vi "LabVIEW RFID.vi"() -> ()   [LabVIEW 2010]
uses:
  <vilib>/Instr/_visa.llb/VISA Configure Serial Port (Instr).vi
  <vilib>/Utility/file.llb/Read From Spreadsheet File (I64).vi
  <vilib>/Utility/file.llb/Read From Spreadsheet File (string).vi
  <vilib>/Utility/file.llb/Write To Spreadsheet File (string).vi
  <vilib>/Utility/file.llb/Write To Spreadsheet File (I64).vi
panel:
  out "var":bool
  in  "Abrir Cacifo a partir de PC":bool
  in  "Endereço de Cacifo a abrir a partir de PC":dbl
  in  "Inserir novo utilizador/dar acesso a cacifo e atualizar base de dados":bool
  in  "default (0 I32)":u64
  in  "Pessoa a retirar acesso":string
  in  "Retirar acesso a cacifo e atualizar base de dasos":bool
  out "Enviado":string
  in  "Endereço do Cacifo a adicionar/remover":dbl
  out "Nomes":string[][](array[string])
  in  "Nome do novo utilizador":string
  out "Qual o utilizador?":string
  out "Código recebido":string
  out "Envia quando encontra 'a'":string
  out "Base de dados":i64[][](array[numeric])
  out "Matriz 2D":i64[][](array[numeric])
  out "Endereço do cacifo":u64
  out "Número de série do cartão":u64
  in  "VISA Resource Name":refnum<visa-resource-name>
  in  "stop":bool
  # "Adicionar utilizador e dar acesso a cacifos"
  # "Dados Recebidos na Porta Série"
  # "Retirar acesso de um utilizador a determinado cacifo"
  # "Reconhecimento de utilizador"
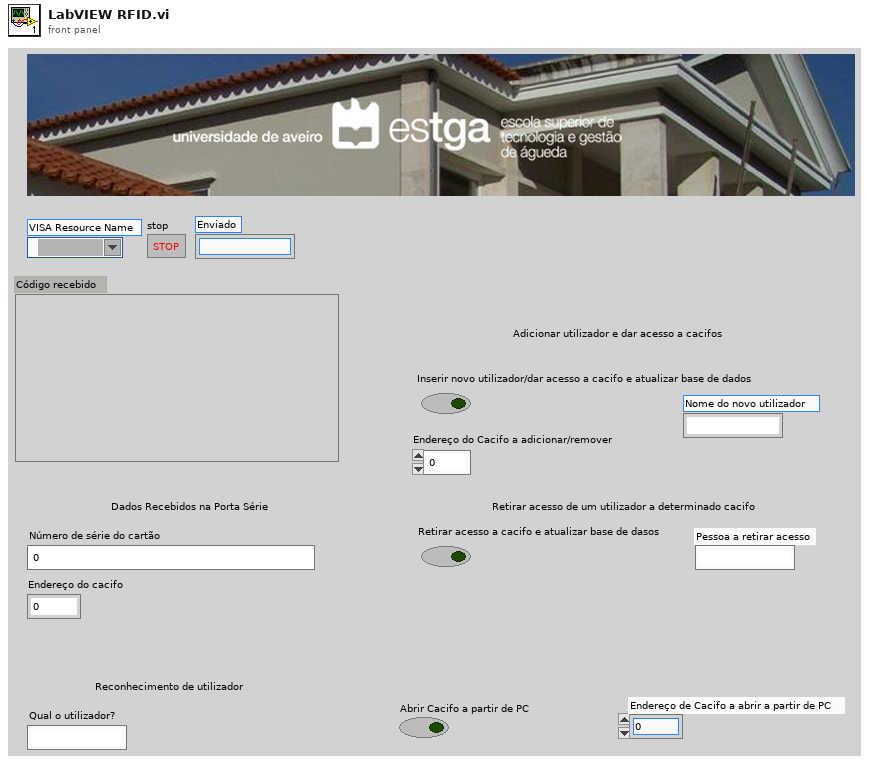
[diagram p1: front panel]
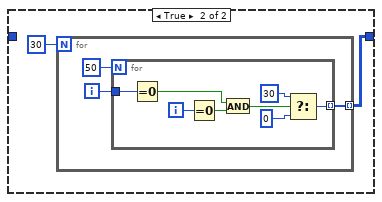
[diagram p3: hidden frame]
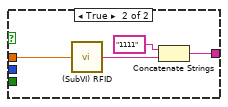
[diagram p4: hidden frame]
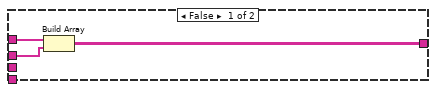
[diagram p6: hidden frame]
diagram:
  w1 = u64 0 ("Endereço do cacifo")
  n1 = local write "Endereço do cacifo"(w1) -> ()
  n2 = local write "Número de série do cartão"(w1) -> ()
  n3 = local write "Envia quando encontra 'a'"("") -> ()
  n4 = call-poly "VISA Configure Serial Port"("VISA resource name"="VISA Resource Name", "Enable Termination\nChar (T)"=FALSE ("Enable Termination\nChar (T)"), "baud rate (9600)"=9600, "data bits (8)"=8, "parity (0:none)"=0) -> ("VISA resource name out"=w8:refnum<visa-resource-name>, "error out"=w7:errorcluster)  [unwired: 9 in]
  n5 = while {
    tunnel: w8 -> [w96]
    tunnel: w7 -> [w95]
    tunnel: [w56] -> w4
    tunnel: [w55] -> w3
    stop <- "stop" stop-if-true
    n6 = flat-sequence {
      tunnel: [w106] -> w81
      tunnel: [w107] -> w80
      tunnel: w95 -> [w101]
      tunnel: w96 -> [w102]
      tunnel: [w99] -> w19
      tunnel: [w120] -> w97
      tunnel: w81 -> [w118]
      tunnel: [w118] -> w85
      tunnel: w80 -> [w117]
      tunnel: [w117] -> w76
      tunnel: w19 -> [w116]
      tunnel: [w116] -> w18
      tunnel: w97 -> [w125]
      tunnel: w85 -> [w133]
      tunnel: [w133] -> w84
      tunnel: w76 -> [w132]
      tunnel: [w132] -> w75
      tunnel: w18 -> [w123]
      tunnel: [w123] -> w13
      tunnel: [w154] -> w94
      tunnel: w84 -> [w152]
      tunnel: [w152] -> w83
      tunnel: [w151] -> w77
      tunnel: w75 -> [w151]
      tunnel: [w150] -> w14
      tunnel: w13 -> [w150]
      tunnel: w94 -> [w180]
      tunnel: [w182] -> w47
      tunnel: [w180] -> w45
      tunnel: [w189] -> w43
      tunnel: [w192] -> w41
      tunnel: [w185] -> w39
      tunnel: ["Nome do novo utilizador"] -> w37
      tunnel: [w186] -> w35
      tunnel: [w184] -> w33
      tunnel: [w183] -> w31
      tunnel: [w180] -> w29
      tunnel: [w179] -> w27
      tunnel: w83 -> [w178]
      tunnel: [w178] -> w25
      tunnel: [w177] -> w23
      tunnel: w77 -> [w177]
      tunnel: [w174] -> w15
      tunnel: w14 -> [w174]
      tunnel: w47 -> [w220]
      tunnel: [w220] -> w46
      tunnel: w45 -> [w219]
      tunnel: [w219] -> w44
      tunnel: w43 -> [w218]
      tunnel: [w218] -> w42
      tunnel: w41 -> [w217]
      tunnel: [w217] -> w40
      tunnel: w39 -> [w216]
      tunnel: [w216] -> w38
      tunnel: w37 -> [w215]
      tunnel: [w215] -> w36
      tunnel: w35 -> [w214]
      tunnel: [w214] -> w34
      tunnel: w33 -> [w213]
      tunnel: [w213] -> w32
      tunnel: w31 -> [w212]
      tunnel: [w212] -> w30
      tunnel: w29 -> [w203]
      tunnel: [w203] -> w28
      tunnel: w27 -> [w202]
      tunnel: [w202] -> w26
      tunnel: w25 -> [w211]
      tunnel: [w211] -> w24
      tunnel: w23 -> [w210]
      tunnel: [w210] -> w22
      tunnel: [w209] -> w21
      tunnel: [w201] -> w16
      tunnel: w15 -> [w201]
      tunnel: w46 -> [w232]
      tunnel: [w232] -> w93
      tunnel: w44 -> [w239]
      tunnel: [w239] -> w92
      tunnel: w42 -> [w238]
      tunnel: [w238] -> w91
      tunnel: w40 -> [w237]
      tunnel: [w237] -> w90
      tunnel: w38 -> [w236]
      tunnel: [w236] -> w89
      tunnel: w36 -> [w235]
      tunnel: [w235] -> w88
      tunnel: w34 -> [w234]
      tunnel: [w234] -> w87
      tunnel: w32 -> [w233]
      tunnel: [w233] -> w86
      tunnel: w30 -> [w228]
      tunnel: w28 -> [_]
      tunnel: w26 -> [_]
      tunnel: w24 -> [w231]
      tunnel: [w231] -> w82
      tunnel: [w230] -> w79
      tunnel: w22 -> [w229]
      tunnel: [w229] -> w78
      tunnel: ["Abrir Cacifo a partir de PC"] -> w69
      tunnel: [w223] -> w67
      tunnel: [w224] -> w63
      tunnel: w21 -> [w223]
      tunnel: ["Abrir Cacifo a partir de PC"] -> w20
      tunnel: [w221] -> w17
      tunnel: w16 -> [w221]
      tunnel: w93 -> [w271]
      tunnel: w92 -> [w275]
      tunnel: w91 -> [w274]
      tunnel: w90 -> [w273]
      tunnel: w89 -> [w266]
      tunnel: w88 -> [w272]
      tunnel: w87 -> [w269]
      tunnel: w86 -> [w265]
      tunnel: w82 -> [w262]
      tunnel: w79 -> [w264]
      tunnel: w78 -> [w263]
      tunnel: [w261] -> w74
      tunnel: [w260] -> w72
      tunnel: [w259] -> w71
      tunnel: w69 -> [_]
      tunnel: w67 -> [w258]
      tunnel: [w258] -> w66
      tunnel: w63 -> [w257]
      tunnel: [w257] -> w62
      tunnel: [w253] -> w59
      tunnel: [w256] -> w56
      tunnel: [w255] -> w55
      tunnel: w20 -> [w254]
      tunnel: w17 -> [w252]
      tunnel: w74 -> [w328]
      tunnel: [w328] -> w73
      tunnel: w72 -> [w327]
      tunnel: w71 -> [w326]
      tunnel: ["Retirar acesso a cacifo e atualizar base de dasos"] -> w70
      tunnel: w66 -> [w324]
      tunnel: [w324] -> w64
      tunnel: w62 -> [w323]
      tunnel: [w323] -> w60
      tunnel: w59 -> [w322]
      tunnel: [w322] -> w57
      tunnel: w73 -> [w367]
      tunnel: w70 -> [w364]
      tunnel: [w367] -> w68
      tunnel: [w363] -> w65
      tunnel: w64 -> [w363]
      tunnel: [w362] -> w61
      tunnel: w60 -> [w362]
      tunnel: [w361] -> w58
      tunnel: w57 -> [w361]
      tunnel: w68 -> [w380]
      tunnel: w65 -> [w378]
      tunnel: w61 -> [w379]
      tunnel: [w380] -> w54
      tunnel: w58 -> [w372]
      tunnel: [w375] -> w52
      tunnel: [w374] -> w51
      tunnel: w54 -> [w393]
      tunnel: [w393] -> w53
      tunnel: w52 -> [w391]
      tunnel: w51 -> [w392]
      tunnel: [w392] -> w50
      tunnel: [w386] -> w49
      tunnel: [w385] -> w48
      tunnel: w53 -> [w411]
      tunnel: w50 -> [w410]
      tunnel: [w411] -> _
      tunnel: w49 -> [w408]
      tunnel: w48 -> [w409]
      frame #0 {
        n7 = property class="Instr"(reference=w102, error in=w101) -> (reference out=w104:refnum<visa-resource-name>, error out=w105:errorcluster, "Serial Settings:Number of Bytes at Serial Port"=w100:u32)
        n8 = Greater?(x=w100, y=46.0 ("x")) -> (0:w99:bool)
        n9 = case shown="True" w99 {
          tunnel: [w108 w115] -> w106
          tunnel: [w109 w114] -> w107
          tunnel: w105 -> [w108 w113]
          tunnel: w104 -> [w109 w112]
          tunnel: w100 -> [_ w111]
          frame False {
          }
          frame True {
            # "(está escondido)"
            n10 = VISA Read(VISA resource name=w112, byte count=w111, error in (no error)=w113) -> (VISA resource name out=w114:refnum<visa-resource-name>, read buffer=→"Código recebido" →"Envia quando encontra 'a'":string, error out=w115:errorcluster)  [unwired: 1 out]
          }
        }
      }
      frame #1 {
        w122 = ""
        n11 = local read "Envia quando encontra 'a'"() -> (w119:string)
        n12 = Equal?(x=w119, y=w122) -> (x = y?=w121:bool)
        n13 = Select(t=w122, s=w121, f=w119) -> (s? t:f=w120:string)
      }
      frame #2 {
        # "Código para obter Número de Série"
        # "Código para obter Endereço do Cacifo"
        n14 = Reverse String(1:w125) -> (0:w124:string)
        n15 = for {
          N: 32 -> [_]
          tunnel: w124 -> [w140]
          tunnel: [w137] -> w127 mode=indexing
          i -> [w136]
          n16 = Add(x=w136, y=7) -> (x+y=w134:i32)
          n17 = String Subset(string=w140, offset (0)=w134, length (rest)=1 ("length (rest)")) -> (substring=w139:string)
          n18 = Equal?(x="1", y=w139) -> (x = y?=w137:bool)
        }
        n19 = for {
          N: 8 -> [_]
          tunnel: w124 -> [w148]
          tunnel: [w145] -> w126 mode=indexing
          i -> [w144]
          n20 = Add(x=39, y=w144) -> (x+y=w142:i32)
          n21 = String Subset(string=w148, offset (0)=w142, length (rest)=1 ("length (rest)")) -> (substring=w147:string)
          n22 = Equal?(x="1", y=w147) -> (x = y?=w145:bool)
        }
        n23 = Boolean Array To Number(Boolean array=w127) -> (number=→"Número de série do cartão":u32)
        n24 = Boolean Array To Number(Boolean array=w126) -> (number=→"Endereço do cacifo":u32)
      }
      frame #3 {
        w156 = 0 ("index")
        n25 = call-poly <vilib>:"Read From Spreadsheet File.vi"("file path (dialog if empty)"=path "C:/Users/rPINA/Dropbox/Projeto temático em Instrumentação Industrial/TesteS de LabVIEW/21-06-2012/Acessos a cacifos.txt" ("new file path (Not A Path if cancelled)")) -> ("all rows"=w155:i64[][])  [unwired: 6 in, 4 out]
        n26 = Index Array(array=w155, index (row)=w156, index (col)=w156) -> (element=w158:i64)
        n27 = Not Equal?(x=w158, y=i64 30) -> (x != y?=w157:bool)
        n28 = case shown="False" w157 {
          tunnel: [w160 w161] -> w154
          tunnel: w155 -> [w160 _]
          frame False {
          }
          frame True {
            n29 = for {
              N: 30 -> [_]
              tunnel: [w163] -> w161 mode=indexing
              i -> [w164]
              n30 = for {
                N: 50 -> [_]
                tunnel: w164 -> [w170]
                tunnel: [w167] -> w163 mode=indexing
                i -> [w173]
                n31 = Equal To 0?(x=w170) -> (x = 0?=w171:bool)
                n32 = Equal To 0?(x=w173) -> (x = 0?=w169:bool)
                n33 = And(x=w171, y=w169) -> (x .and. y?=w172:bool)
                n34 = Select(t=u64 30, s=w172, f=u64 0) -> (s? t:f=w167:u64)
              }
            }
          }
        }
        "Matriz 2D" <- w154
      }
      frame #4 {
        w181 = -1 ("y")
        n35 = local read "Endereço do Cacifo a adicionar/remover"() -> (w187:dbl)
        n36 = local read "Número de série do cartão"() -> (w179:u64)
        n37 = Increment(x=w187) -> (x+1=w200:dbl)
        n38 = Index Array(array=w180, index (row)=w200) -> (element=w199:u64[])  [unwired: 1 in]
        n39 = call-poly <vilib>:"Read From Spreadsheet File.vi"("file path (dialog if empty)"=path "C:/Users/rPINA/Dropbox/Projeto temático em Instrumentação Industrial/TesteS de LabVIEW/21-06-2012/Nomes e numeros de série.txt") -> ("all rows"=w194:string[][])  [unwired: 6 in, 4 out]
        n40 = Search 1D Array(1D array=w199, element=w179) -> (index of element=w198:i32)  [unwired: 1 in]
        n41 = Number To Decimal String(number=w179) -> (decimal integer string=w195:string)  [unwired: 1 in]
        n42 = Index Array(array=w194, index (row)=1) -> (element=w192:string[])  [unwired: 1 in]
        n43 = Equal?(x=w198, y=w181) -> (x = y?=w182:bool)
        n44 = Search 1D Array(1D array=w192, element=w195) -> (index of element=w191:i32)  [unwired: 1 in]
        n45 = Index Array(array=w194, index (row)=0) -> (element=w189:string[])  [unwired: 1 in]
        n46 = Equal?(x=w191, y=w181) -> (x = y?=w185:bool)
        n47 = Search 1D Array(1D array=w189, element="Nome do novo utilizador") -> (index of element=w188:i32)  [unwired: 1 in]
        n48 = Index Array(array=w189, index=w191) -> (element=→"Qual o utilizador?":string)
        n49 = local read "Endereço do cacifo"() -> (w183:u64)
        n50 = Equal?(x=w188, y=w181) -> (x = y?=w186:bool)
        n51 = Equal?(x=w183, y=u32 1) -> (x = y?=w184:bool)
      }
      frame #5 {
        n52 = local read "Endereço do cacifo"() -> (w205:u64)
        n53 = Increment(x=w205) -> (x+1=w204:u64)
        n54 = Index Array(array=w203, index (row)=w204) -> (element=w206:u64[])  [unwired: 1 in]
        n55 = Search 1D Array(1D array=w206, element=w202) -> (index of element=w208:i32)  [unwired: 1 in]
        n56 = Equal?(x=w208, y=-1 ("start index (0)")) -> (x = y?=w209:bool)
      }
      frame #6 {
        n57 = Less Or Equal?(x="Endereço de Cacifo a abrir a partir de PC", y=u32 255) -> (x <= y?=w226:bool)
        n58 = And(x="Abrir Cacifo a partir de PC", y=w226) -> (x .and. y?=w224:bool)
        n59 = case shown="False" w224 {
          tunnel: w223 -> [w243 _]
          tunnel: [w242 w249] -> w230
          tunnel: w228 -> [w244 _]
          tunnel: "Endereço de Cacifo a abrir a partir de PC" -> [_ w250]
          frame False {
            n60 = call "(SubVI) RFID.vi"("Nº Decimal"=w244) -> ("Nº Binário"=w245:string)
            n61 = Concatenate Strings("0000" ("f"), w245) -> (w246:string)
            n62 = Concatenate Strings("1111", w245) -> (w247:string)
            n63 = Select(t=w246, s=w243, f=w247) -> (s? t:f=w242:string)
          }
          frame True {
            n64 = call "(SubVI) RFID.vi"("Nº Decimal"=w250) -> ("Nº Binário"=w248:string)
            n65 = Concatenate Strings("1111", w248) -> (w249:string)
          }
        }
        "Enviado" <- w230
      }
      frame #7 {
        n66 = Not(x=w266) -> (.not. x?=w267:bool)
        n67 = Or(x=w254, y=w252) -> (x .or. y?=w253:bool)
        n68 = Compound Arithmetic op=AND(w269, w266, w265) -> (w268:bool)
        n69 = case shown="True" w268 {
          tunnel: w274 -> [w294 w303]
          tunnel: w273 -> [_ w302]
          tunnel: [w292 w296] -> w260
          tunnel: w273 -> [w293 _]
          tunnel: w272 -> [_ w295]
          frame False {
            n70 = Build Array(w294, w293) -> (w292:string[][])
          }
          frame True {
            n71 = local read "Número de série do cartão"() -> (w301:u64)
            n72 = Number To Decimal String(number=w301) -> (decimal integer string=w300:string)  [unwired: 1 in]
            n73 = Insert Into Array(array=w303, index=0, new element=w295) -> (w298:string[])
            n74 = Insert Into Array(array=w302, index=0, new element=w300) -> (w297:string[])
            n75 = Build Array(w298, w297) -> (w296:string[][])
          }
        }
        "Nomes" <- w260
        n76 = Compound Arithmetic op=AND(w271, w265, w267) -> (w270:bool)
        n77 = case shown="True" w270 {
          tunnel: w275 -> [w305 w308]
          tunnel: [w305 w307] -> w259
          frame False {
          }
          frame True {
            n78 = local read "Endereço do Cacifo a adicionar/remover"() -> (w306:dbl)
            n79 = Increment(x=w306) -> (x+1=w310:dbl)
            n80 = local read "Número de série do cartão"() -> (w318:u64)
            n81 = Index Array(array=w308, index (row)=w310) -> (element=w317:u64[])  [unwired: 1 in]
            n82 = Index Array(array=w317, index=u64 0 ("element")) -> (element=w320:u64)
            n83 = Increment(x=w320) -> (x+1=w319:u64)
            n84 = Replace Array Subset(array=w317, new element=w318, index=w319) -> (w312:u64[])
            n85 = Index Array(array=w312, index=0) -> (element=w316:u64)
            n86 = Increment(x=w316) -> (x+1=w314:u64)
            n87 = local read "Matriz 2D"() -> (w311:i64[][])
            n88 = Replace Array Subset(array=w312, new element=w314, index=0) -> (w309:u64[])
            n89 = Replace Array Subset(array=w311, new element=w309, index (row)=w310) -> (w307:i64[][])  [unwired: 1 in]
          }
        }
        "Base de dados" <- w259
        n90 = case shown="True" w253 {
          tunnel: [w276 w283] -> w255
          tunnel: [w277 w282] -> w256
          tunnel: w264 -> [_ w280]
          tunnel: w263 -> [w277 w279]
          tunnel: w262 -> [w276 w278]
          frame False {
          }
          frame True {
            n91 = String Length(string=w280) -> (length=w281:i32)
            n92 = for {
              N: w281 -> [_]
              tunnel: [w291] -> w283
              tunnel: [w290] -> w282
              tunnel: w280 -> [w289]
              tunnel: w279 -> [w286]
              tunnel: w278 -> [w285]
              i -> [w284]
              n93 = String Subset(string=w289, offset (0)=w284, length (rest)=1 ("length (rest)")) -> (substring=w288:string)
              n94 = VISA Write(VISA resource name=w286, write buffer=w288, error in (no error)=w285) -> (VISA resource name out=w290:refnum<visa-resource-name>, error out=w291:errorcluster)  [unwired: 1 out]
            }
          }
        }
        n95 = local read "Enviado"() -> (w261:string)
      }
      frame #8 {
        n96 = case shown="True" "Retirar acesso a cacifo e atualizar base de dasos" {
          tunnel: w327 -> [_ w349]
          tunnel: w326 -> [_ w336]
          frame False {
          }
          frame True {
            w333 = 0 ("index")
            n97 = local read "Endereço do Cacifo a adicionar/remover"() -> (w335:dbl)
            n98 = Index Array(array=w349, index (row)=0) -> (element=w347:string[])  [unwired: 1 in]
            n99 = Search 1D Array(1D array=w347, element="Pessoa a retirar acesso") -> (index of element=w343:i32)  [unwired: 1 in]
            n100 = Index Array(array=w349, index (row)=1) -> (element=w344:string[])  [unwired: 1 in]
            n101 = Index Array(array=w344, index=w343) -> (element=w342:string)
            n102 = Decimal String To Number(string=w342, default (0L)="default (0 I32)") -> (number=w339:u64)  [unwired: 1 in, 1 out]
            n103 = Increment(x=w335) -> (x+1=w334:dbl)
            n104 = Index Array(array=w336, index (row)=w334) -> (element=w340:u64[])  [unwired: 1 in]
            n105 = Index Array(array=w340, index=w333) -> (element=w337:u64)
            n106 = Replace Array Subset(array=w340, new element=w333, index=w333) -> (w338:u64[])
            n107 = Decrement(x=w337) -> (x-1=w332:u64)
            n108 = Search 1D Array(1D array=w338, element=w339) -> (index of element=w331:i32)  [unwired: 1 in]
            n109 = Not Equal?(x=w331, y=-1.0) -> (x != y?=w329:bool)
            n110 = case shown="True" w329 {
              tunnel: w338 -> [_ w360]
              tunnel: w331 -> [_ w359]
              tunnel: w336 -> [_ w358]
              tunnel: w334 -> [_ w357]
              tunnel: w333 -> [_ w353]
              tunnel: w332 -> [_ w352]
              frame False {
              }
              frame True {
                n111 = Replace Array Subset(array=w360, new element=w353, index=w359) -> (w356:u64[])
                n112 = Sort 1D Array(array=w356) -> (sorted array=w355:u64[])
                n113 = Reverse 1D Array(array=w355) -> (reversed array=w354:u64[])
                n114 = Insert Into Array(array=w354, index=w353, new element=w352) -> (w351:u64[])
                n115 = Replace Array Subset(array=w358, new element=w351, index (row)=w357) -> (w350:u64[][])  [unwired: 1 in]
                n116 = local write "Base de dados"(w350) -> ()
              }
            }
          }
        }
      }
      frame #9 {
        n117 = Or(x="Inserir novo utilizador/dar acesso a cacifo e atualizar base de dados", y=w364) -> (x .or. y?=w365:bool)
        n118 = case shown="True" w365 {
          frame False {
          }
          frame True {
            n119 = local read "Base de dados"() -> (w368:i64[][])
            n120 = local read "Nomes"() -> (w370:string[][])
            n121 = call-poly <vilib>:"Write To Spreadsheet File.vi"("2D data"=w368, "file path (dialog if empty)"=path "C:/Users/rPINA/Dropbox/Projeto temático em Instrumentação Industrial/TesteS de LabVIEW/02-07-2012/Acessos a cacifos.txt" ("new file path (Not A Path if cancelled)")) -> ()  [unwired: 6 in, 1 out]
            n122 = call-poly <vilib>:"Write To Spreadsheet File.vi"("2D data"=w370, "file path (dialog if empty)"=path "C:/Users/rPINA/Dropbox/Projeto temático em Instrumentação Industrial/TesteS de LabVIEW/02-07-2012/Nomes e numeros de série.txt") -> ()  [unwired: 6 in, 1 out]
          }
        }
      }
      frame #10 {
        # "Evitar probema de guardar endereço 0 no ficheiro"
        n123 = local read "Endereço do cacifo"() -> (w375:u64)
        n124 = Not Equal To 0?(x=w375) -> (x != 0?=w373:bool)
        n125 = Not(x=w379) -> (.not. x?=w376:bool)
        n126 = Not(x=w378) -> (.not. x?=w377:bool)
        n127 = Compound Arithmetic op=AND(w376, w377, w373, w372) -> (w374:bool)
        "var" <- w374
      }
      frame #11 {
        n128 = local read "Qual o utilizador?"() -> (w382:string)
        n129 = Number To Decimal String(number=w391) -> (decimal integer string=w387:string)  [unwired: 1 in]
        n130 = String Length(string=w382) -> (length=w383:i32)
        n131 = String Length(string=w387) -> (length=w389:i32)
        n132 = Subtract(x=20.0, y=w383) -> (x-y=w381:dbl)
        n133 = Subtract(x=20.0, y=w389) -> (x-y=w388:dbl)
        n134 = for {
          N: w381 -> [_]
          shift-right: [w394] -> _
          shift-left: _ -> [w395]
          tunnel: w382 -> [w397]
          tunnel: [w394] -> w385
          i -> [w398]
          n135 = Equal To 0?(x=w398) -> (x = 0?=w399:bool)
          n136 = Select(t=w397, s=w399, f=w395) -> (s? t:f=w396:string)
          n137 = call <vilib>:"Space Constant.vi"() -> ("String"=w400:string)
          n138 = Concatenate Strings(w396, w400) -> (w394:string)
        }
        n139 = for {
          N: w388 -> [_]
          shift-right: [w401] -> _
          shift-left: _ -> [w402]
          tunnel: w387 -> [w404]
          tunnel: [w401] -> w386
          i -> [w405]
          n140 = Equal To 0?(x=w405) -> (x = 0?=w406:bool)
          n141 = Select(t=w404, s=w406, f=w402) -> (s? t:f=w403:string)
          n142 = call <vilib>:"Space Constant.vi"() -> ("String"=w407:string)
          n143 = Concatenate Strings(w403, w407) -> (w401:string)
        }
      }
      frame #12 {
        n144 = case shown="True" w410 {
          tunnel: w409 -> [_ w417]
          tunnel: w408 -> [_ w416]
          frame False {
          }
          frame True {
            w424 = path "C:/Users/rPINA/Dropbox/Projeto temático em Instrumentação Industrial/TesteS de LabVIEW/02-07-2012/Registos de acessos com horas.txt" ("new file path (Not A Path if cancelled)")
            w426 = 0 ("index (row)")
            w432 = 0 ("index")
            n145 = local write "var"(FALSE) -> ()
            n146 = Get Date/Time In Seconds() -> (seconds since 1Jan1904=w431:timestamp)
            n147 = Format Date/Time String(time format string (%c)="%H", seconds (now)=w431) -> (date/time string=w437:string)  [unwired: 1 in]
            n148 = Format Date/Time String(time format string (%c)="%M", seconds (now)=w431) -> (date/time string=w436:string)  [unwired: 1 in]
            n149 = Format Date/Time String(time format string (%c)="%S", seconds (now)=w431) -> (date/time string=w435:string)  [unwired: 1 in]
            n150 = Concatenate Strings(w437, "h" ("string")) -> (w444:string)
            n151 = Concatenate Strings(w436, "m" ("string")) -> (w443:string)
            n152 = Format Date/Time String(time format string (%c)="%x", seconds (now)=w431) -> (date/time string=w414:string)  [unwired: 1 in]
            n153 = Concatenate Strings(w435, "s" ("string")) -> (w441:string)
            n154 = call <vilib>:"Space Constant.vi"() -> ("String"=w413:string)
            n155 = call <vilib>:"Space Constant.vi"() -> ("String"=w415:string)
            n156 = call-poly <vilib>:"Read From Spreadsheet File.vi"("file path (dialog if empty)"=w424) -> ("all rows"=w425:string[][])  [unwired: 6 in, 4 out]
            n157 = Concatenate Strings(w414, w413, w413, w413, w413, w413, w413, w413, w413, w413, w413) -> (w412:string)
            n158 = Concatenate Strings(w444, w443, w441, w415, w415, w415, w415, w415, w415, w415, w415, w415, w415, w415) -> (w440:string)
            n159 = Index Array(array=w425, index (row)=w426) -> (element=w427:string[])  [unwired: 1 in]
            n160 = Index Array(array=w425, index (row)=1) -> (element=w428:string[])  [unwired: 1 in]
            n161 = Index Array(array=w425, index (row)=2) -> (element=w438:string[])  [unwired: 1 in]
            n162 = Index Array(array=w425, index (row)=3) -> (element=w433:string[])  [unwired: 1 in]
            n163 = Insert Into Array(array=w427, index=w426, new element=w412) -> (w422:string[])
            n164 = Insert Into Array(array=w428, index=w432, new element=w440) -> (w421:string[])
            n165 = Insert Into Array(array=w438, index=w432, new element=w417) -> (w420:string[])
            n166 = Insert Into Array(array=w433, index=w432, new element=w416) -> (w419:string[])
            n167 = Build Array(w422, w421, w420, w419) -> (w423:string[][])
            n168 = call-poly <vilib>:"Write To Spreadsheet File.vi"("2D data"=w423, "file path (dialog if empty)"=w424) -> ()  [unwired: 6 in, 1 out]
          }
        }
      }
    }
  }
  n169 = VISA Close(VISA resource name=w4, error in (no error)=w3) -> (error out=w5:errorcluster)
  n170 = call <vilib>:"Simple Error Handler.vi"("error in (no error)"=w5) -> ()  [unwired: 4 in, 5 out]
